vi "interp1 (1D).vi"(0 "X":dbl[](array[numeric]), 2 "Y":dbl[](array[numeric]), 3 "U":dbl[](array[numeric]), 4 "extrapolate (T)":bool=TRUE) -> (5 "V":dbl[](array[numeric]))   [LabVIEW 2020]
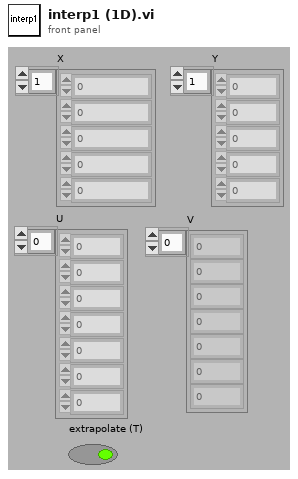
[diagram p1: front panel]
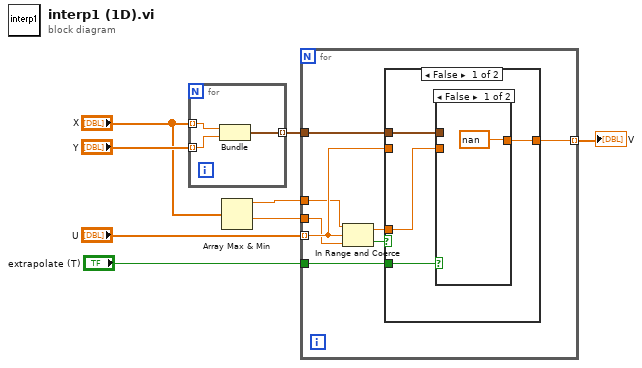
[diagram p0: block diagram]
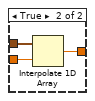
[diagram p2: hidden frame]
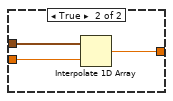
[diagram p3: hidden frame]
diagram:
  n1 = for {
    tunnel: "X" -> [w11] mode=indexing
    tunnel: "Y" -> [w10] mode=indexing
    tunnel: [w9] -> w7 mode=indexing
    n2 = Bundle("Numeric"=w11, "Numeric"=w10) -> (w9:cluster{"Numeric":dbl, "Numeric":dbl})  [unwired: 1 in]
  }
  n3 = Array Max & Min(array="X") -> (max value=w3:dbl, min value=w2:dbl)  [unwired: 2 out]
  n4 = for {
    tunnel: w7 -> [w19]
    tunnel: [w18] -> w5 mode=indexing
    tunnel: "U" -> [w17] mode=indexing
    tunnel: w3 -> [w15]
    tunnel: w2 -> [w16]
    tunnel: "extrapolate (T)" -> [w12]
    n5 = In Range and Coerce(upper limit=w15, x=w17, lower limit=w16) -> (coerced(x)=w13:dbl, In Range?=w14:bool)
    n6 = case shown="False" w14 {
      tunnel: w19 -> [w23 w30]
      tunnel: [w21 w29] -> w18
      tunnel: w17 -> [_ w28]
      tunnel: w13 -> [w22 _]
      tunnel: w12 -> [w20 _]
      frame False {
        n7 = case shown="False" w20 {
          tunnel: w23 -> [_ w27]
          tunnel: w22 -> [_ w26]
          tunnel: [nan w25] -> w21
          frame False {
          }
          frame True {
            n8 = Interpolate 1D Array(1:w26, 2:w27) -> (0:w25:dbl)
          }
        }
      }
      frame True {
        n9 = Interpolate 1D Array(1:w28, 2:w30) -> (0:w29:dbl)
      }
    }
  }
  "V" <- w5
